vi "clock.vi"() -> ()   [LabVIEW 2014]
doc: "This is an example VI which uses four guages to show an analogue clock. The timestamp is retrieved from the computer, and analysed every 100ms. Values for hour, minute, and seconds are single precision, and the clock is updated every 100ms. This gives the impression of constantly flowing dials."
panel:
  out "Second":sgl(knob) scale=0.0..60.0
  out "Minute":sgl(knob) scale=0.0..60.0
  out "Hour":sgl(knob) scale=0.0..12.0
  out "Dial":sgl(knob) scale=0.0..12.0
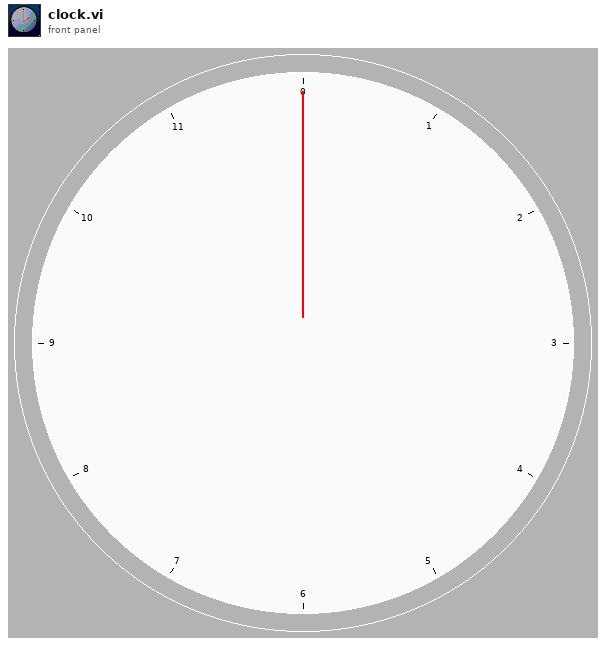
[diagram p1: front panel]
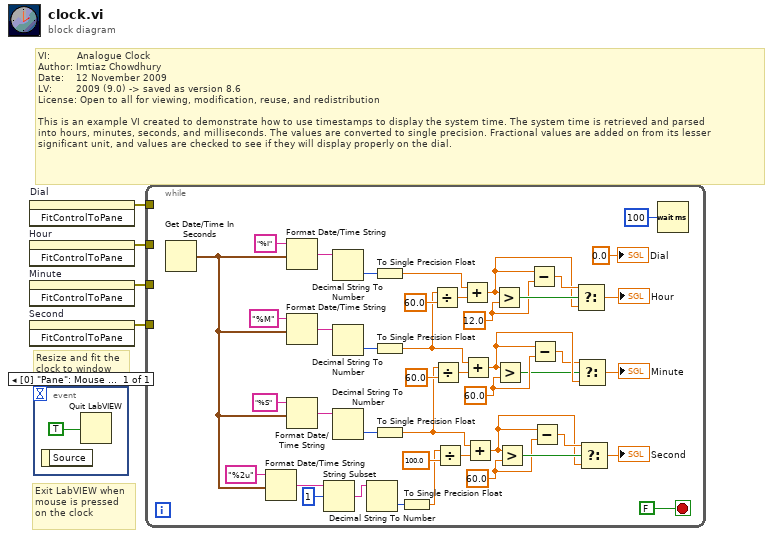
[diagram p0: block diagram]
diagram:
  # "Exit LabVIEW when\nmouse is pressed\non the clock"
  # "Resize and fit the\nclock to window"
  # "VI:         Analogue Clock\nAuthor: Imtiaz Chowdhury\nDate:    12 November 2009\nLV:        2009 (9.0) -> saved as version 8.6\nLicense: Open to all for viewing, modification, reuse, and redistribution\n\nThis is an example VI created to demonstrate how to use timestamps to display the system time. The system time is retrieved and parsed\ninto hours, minutes, seconds, and milliseconds. The values are converted to single precision. Fractional values are added on from its lesser\nsignificant unit, and values are checked to see if they will display properly on the dial."
  n1 = invoke on="Dial" class="Knob (strict)" method="FitControlToPane"() -> (error out=w4:errorcluster)  [unwired: 3 in, 2 out]
  n2 = invoke on="Hour" class="Knob (strict)" method="FitControlToPane"() -> (error out=w3:errorcluster)  [unwired: 3 in, 2 out]
  n3 = invoke on="Minute" class="Knob (strict)" method="FitControlToPane"() -> (error out=w2:errorcluster)  [unwired: 3 in, 2 out]
  n4 = invoke on="Second" class="Knob (strict)" method="FitControlToPane"() -> (error out=w1:errorcluster)  [unwired: 3 in, 2 out]
  n5 = event shown="[0] \"Pane\": Mouse Down" {
    selector: _ -> [_]
    dyn-events: _ -> [_]
    timeout: _ -> [_]
    event Mouse Down {
      n6 = event-data() -> ()  [unwired: 1 in, 1 out]
      n7 = Quit LabVIEW(quit? (T)=TRUE) -> ()
    }
  }
  n8 = while {
    tunnel: w4 -> [_]
    tunnel: w3 -> [_]
    tunnel: w2 -> [_]
    tunnel: w1 -> [_]
    stop <- FALSE stop-if-true
    w12 = sgl 60.0 ("y")
    w27 = sgl 60.0 ("y")
    w32 = sgl 12.0 ("y")
    n9 = Get Date/Time In Seconds() -> (seconds since 1Jan1904=w20:timestamp)
    n10 = Format Date/Time String(time format string (%c)="%2u", seconds (now)=w20) -> (date/time string=w19:string)  [unwired: 1 in]
    n11 = Format Date/Time String(time format string (%c)="%I", seconds (now)=w20) -> (date/time string=w44:string)  [unwired: 1 in]
    n12 = Format Date/Time String(time format string (%c)="%M", seconds (now)=w20) -> (date/time string=w41:string)  [unwired: 1 in]
    n13 = Format Date/Time String(time format string (%c)="%S", seconds (now)=w20) -> (date/time string=w39:string)  [unwired: 1 in]
    n14 = String Subset(string=w19, offset (0)=1) -> (substring=w16:string)  [unwired: 1 in]
    n15 = Decimal String To Number(string=w44) -> (number=w43:i32)  [unwired: 2 in, 1 out]
    n16 = Decimal String To Number(string=w41) -> (number=w42:i32)  [unwired: 2 in, 1 out]
    n17 = Decimal String To Number(string=w39) -> (number=w40:i32)  [unwired: 2 in, 1 out]
    n18 = Decimal String To Number(string=w16) -> (number=w17:i32)  [unwired: 2 in, 1 out]
    n19 = To Single Precision Float(number=w43) -> (single precision float=w35:sgl)
    n20 = To Single Precision Float(number=w42) -> (single precision float=w23:sgl)
    n21 = To Single Precision Float(number=w40) -> (single precision float=w9:sgl)
    n22 = To Single Precision Float(number=w17) -> (single precision float=w8:sgl)
    n23 = Divide(x=w23, y=sgl 60.0) -> (x/y=w37:sgl)
    n24 = Divide(x=w9, y=sgl 60.0) -> (x/y=w24:sgl)
    n25 = Divide(x=w8, y=sgl 100.0) -> (x/y=w15:sgl)
    n26 = Add(x=w35, y=w37) -> (x+y=w30:sgl)
    n27 = Add(x=w23, y=w24) -> (x+y=w29:sgl)
    n28 = Add(x=w9, y=w15) -> (x+y=w10:sgl)
    n29 = Greater?(x=w30, y=w32) -> (0:w34:bool)
    n30 = Greater?(x=w29, y=w27) -> (0:w26:bool)
    n31 = Greater?(x=w10, y=w12) -> (0:w13:bool)
    n32 = Subtract(x=w30, y=w32) -> (x-y=w31:sgl)
    n33 = Subtract(x=w29, y=w27) -> (x-y=w28:sgl)
    n34 = Subtract(x=w10, y=w12) -> (x-y=w11:sgl)
    n35 = Select(t=w31, s=w34, f=w30) -> (s? t:f=→"Hour":sgl)
    n36 = Select(t=w28, s=w26, f=w29) -> (s? t:f=→"Minute":sgl)
    n37 = Select(t=w11, s=w13, f=w10) -> (s? t:f=→"Second":sgl)
    n38 = Wait (ms)(milliseconds to wait=u32 100 ("millisecond multiple")) -> ()  [unwired: 1 out]
    "Dial" <- sgl 0.0 ("Dial")
  }
